vi "5RobotsTactic.vi"(5 "firstCall":bool, 8 "error in (no error)":errorcluster, 9 "Robot In":refnum<class "Robot.lvclass">, 10 "Game in":refnum<class "Game.lvclass">, 11 "5RobotsTactic in":refnum<class "5RobotsTactic.lvclass">) -> (0 "error out":errorcluster, 2 "Robot out":refnum<class "Robot.lvclass">, 3 "5RobotsTactic out":refnum<class "5RobotsTactic.lvclass">)   [LabVIEW 2023, in "5RobotsTactic.lvclass"]
uses:
  5RobotsTactic.lvclass
  C:/Users/ebert/Desktop/roboime/SSL_AI/Tactic_class/Tactic.lvclass
  Robot_class/Robot.lvclass
  Game_class/Game.lvclass
  Robot_class/tactics.ctl
  Tactic_class/Tactic.lvclass/Tactic.ctl
  Robot_class/Robot.lvclass/Robot.ctl
  Tactic_class/Read Skillbook.vi
  Robot_class/Write tactic.vi
  Robot_class/Write keepDest.vi
  Skillbook_class/Skillbook.lvclass
  5RobotsSkill_class/5RobotsSkill.lvclass
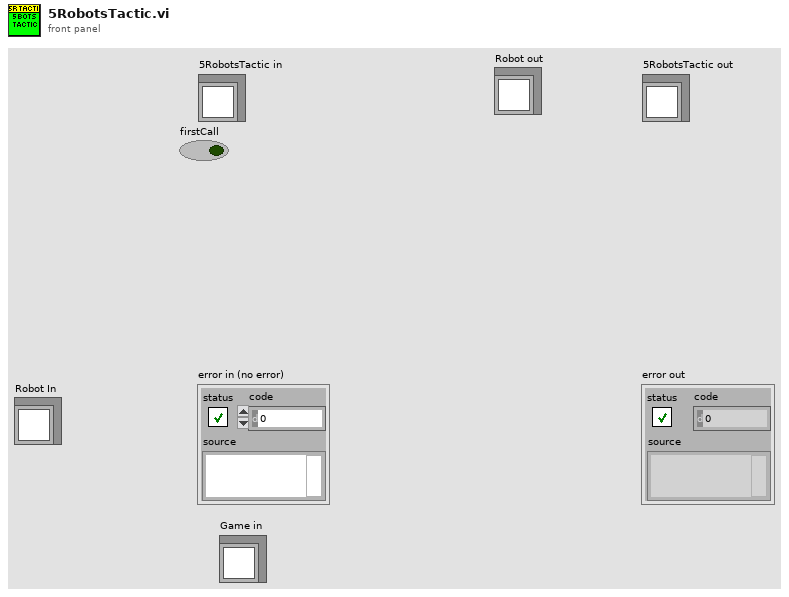
[diagram p1: front panel]
types:
  T1 = typedef "tactics.ctl" = enum16{"GoToBallPlacementPosition", "PlaceBall", "GoToBallPlacement", "5Robots", "BallPlacementEnemy", "ReceivePassInFuturePoint", "Roller", "PrepareRollToPassRollerGoTo", "PrepareRollToPassReceiverGoTo", "WaitRoll", "PositionToRoll", "PenaltyAttacker", "PassObserver", "PenaltyDefense", "TableReceiverTactic", "Test", "DefendGoal", "Marker", "FollowAttacker", "DefendArea", "Shoot", "AttackerAimGoal", "AttackerBallOutOfField", "AttackerBlock", "AttackerStop", "Duelist", "Halt", "ZigZag", "GoTo", "Timeout", "KickToBestRobot", "KickToPassReceiver", "PositionToReceivePass", "WaitPass", "GoToTarget"}
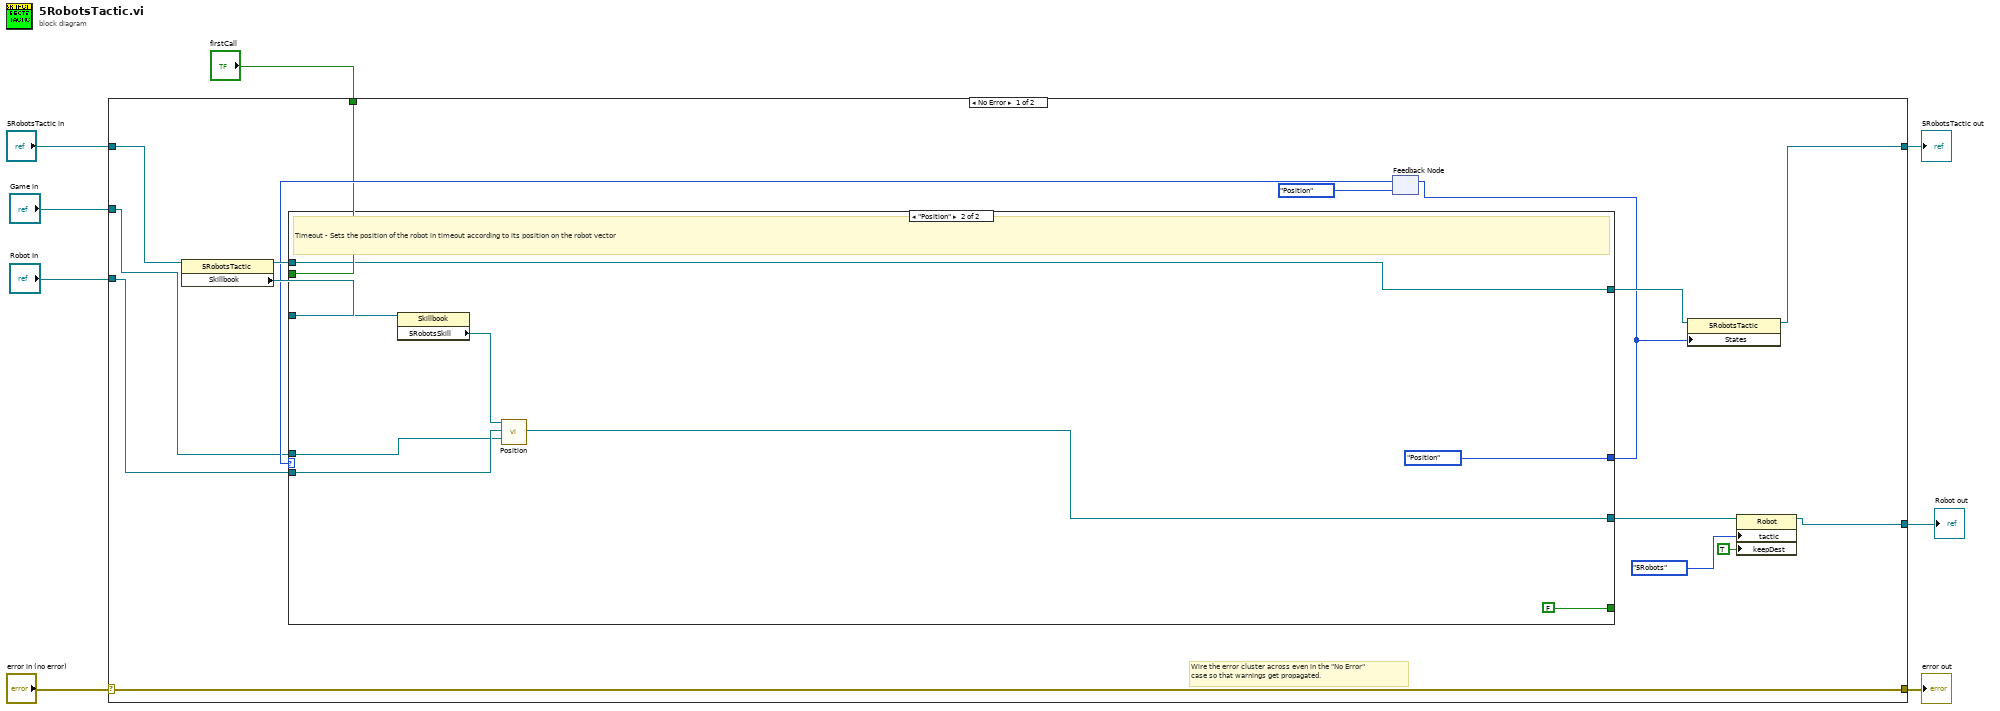
[diagram p0: block diagram]
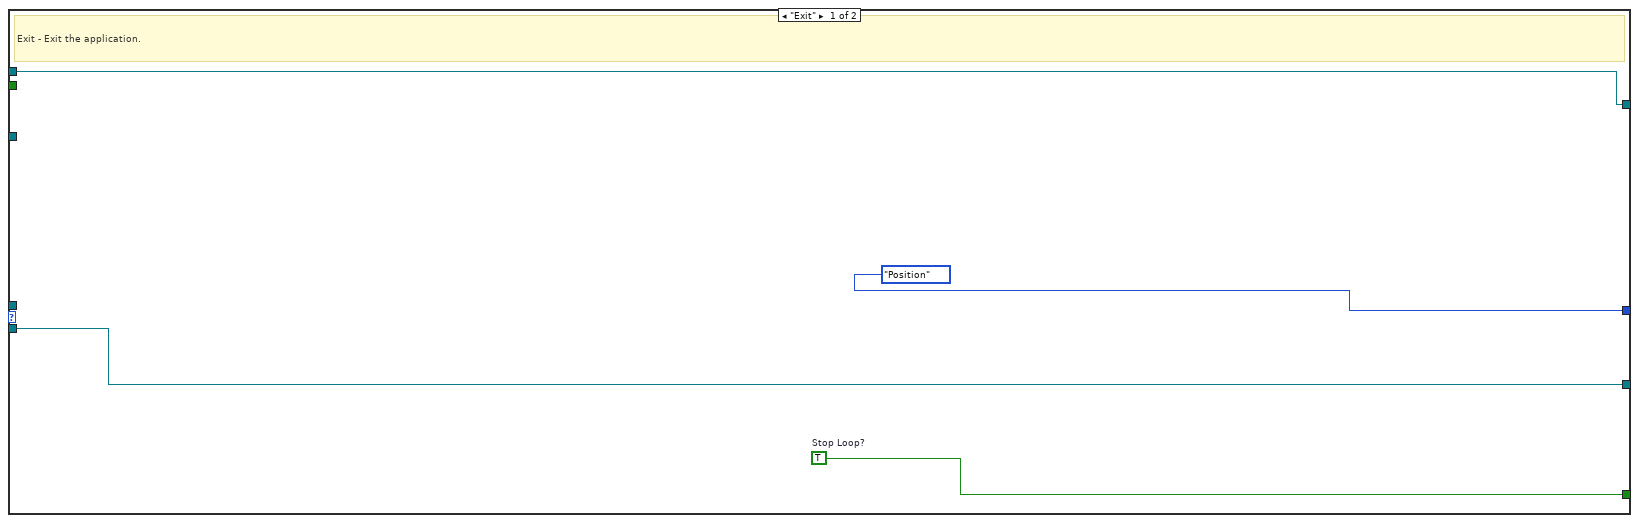
[diagram p2: hidden frame]
diagram:
  n1 = case shown="No Error" "error in (no error)" {
    selector: "error in (no error)" -> [w24 w39]
    tunnel: [w24 w39] -> w7
    tunnel: [w15 w38] -> w5
    tunnel: "5RobotsTactic in" -> [w23 w38]
    tunnel: [w16 w37] -> w4
    tunnel: "Robot In" -> [w12 w37]
    tunnel: "Game in" -> [w13 _]
    tunnel: "firstCall" -> [w11 _]
    frame No Error {
      # "Wire the error cluster across even in the \"No Error\"\ncase so that warnings get propagated."
      n2 = property class="5RobotsTactic"(reference=w23) -> (reference out=w20:refnum<class "5RobotsTactic.lvclass">, "Skillbook"=w22:refnum<class "Skillbook.lvclass">)  [unwired: 1 in, 1 out]
      n3 = feedback #1(enum16{"Position", "Exit"}."Position" ("States")) -> (w19:enum16{"Position", "Exit"})
      n4 = case shown="\"Position\"" w19 {
        tunnel: [w28 FALSE ("Stop Loop?")] -> _
        tunnel: w22 -> [_ w35]
        tunnel: [w25 w34] -> w21
        tunnel: w20 -> [w25 w34]
        tunnel: [enum16{"Position", "Exit"}."Position" ("States") enum16{"Position", "Exit"}."Position" ("States")] -> w10
        tunnel: [w26 w29] -> w14
        tunnel: w13 -> [_ w30]
        tunnel: w12 -> [w26 w32]
        tunnel: w11 -> [_ _]
        frame "Exit" {
          w28 = TRUE  # Stop Loop?
          # "Exit - Exit the application."
        }
        frame "Position" {
          # "Timeout - Sets the position of the robot in timeout according to its position on the robot vector"
          n5 = property class="Skillbook"(reference=w35) -> ("5RobotsSkill"=w31:refnum<class "5RobotsSkill.lvclass">)  [unwired: 1 in, 2 out]
          n6 = call-dynamic "Position.vi"("object in"=w31, "Robot"=w32, "Game"=w30) -> ("Robot out"=w29:refnum<class "Robot.lvclass">)  [unwired: 14 in, 2 out]
        }
      }
      n7 = feedback-in #1(w10) -> ()
      n8 = property class="5RobotsTactic"(reference=w21, "States"=w10) -> (reference out=w15:refnum<class "5RobotsTactic.lvclass">)  [unwired: 1 in, 1 out]
      n9 = property class="Robot"(reference=w14, "tactic"=tactics."5Robots", "keepDest"=TRUE) -> (reference out=w16:refnum<class "Robot.lvclass">)  [unwired: 1 in, 1 out]
    }
    frame Error {
    }
  }
  "error out" <- w7
  "5RobotsTactic out" <- w5
  "Robot out" <- w4
